vi "Send NEA_Get Data.vi"(7 "Message Priority (Normal)":T2=enum."Normal", 8 "error in (no error)":errorcluster, 10 "Data":T1={"M2 Dataset"={"Read Temp"=273.15, "Feedback"=1, "Set Temp"=273.15}, "M1 Dataset"={"Read Temp"=273.15, "Feedback"=1, "Set Temp"=273.15}, "Comp"=FALSE} {"M1 Dataset"."Set Temp" format="%.1f"; "M1 Dataset"."Feedback" items=["Evap Temp", "Case Temp", "Intec Temp", "TSD  Temp", "Autotune", "Extra"]; "M1 Dataset"."Read Temp" format="%.1f"; "M2 Dataset"."Set Temp" format="%.1f"; "M2 Dataset"."Feedback" items=["Evap Temp", "Case Temp", "Intec Temp", "TSD  Temp", "Autotune", "Extra"]; "M2 Dataset"."Read Temp" format="%.1f"}, 11 "Message Enqueuer":refnum<class "Message Enqueuer.lvclass">) -> (0 "error out":errorcluster, 3 "Message Enqueuer out":refnum<class "Message Enqueuer.lvclass">)   [LabVIEW 2019, in "Test.lvlib" / "NEA_Get Data Msg.lvclass"]
doc: "This VI sends the message to an actor."
uses:
  NEA_Get Data Msg.lvclass
  <vilib>/ActorFramework/Message Enqueuer/Message Enqueuer.lvclass
  <vilib>/ActorFramework/Message Enqueuer/Message Priority.ctl
  Type Defs/Cobra Data.ctl
  C:/Program Files (x86)/National Instruments/LabVIEW 2019/vi.lib/ActorFramework/Message/Message.lvclass
  NEA_Get Data Msg.lvclass/NEA_Get Data Msg.ctl
  <vilib>/ActorFramework/Message Enqueuer/Message Enqueuer.lvclass/Message Enqueuer.ctl
  <vilib>/ActorFramework/Message Priority Queue/Priority Enqueue.vi
  Test.lvlib
panel:
  # "degC"
  # "degC"
  # "degC"
  # "degC"
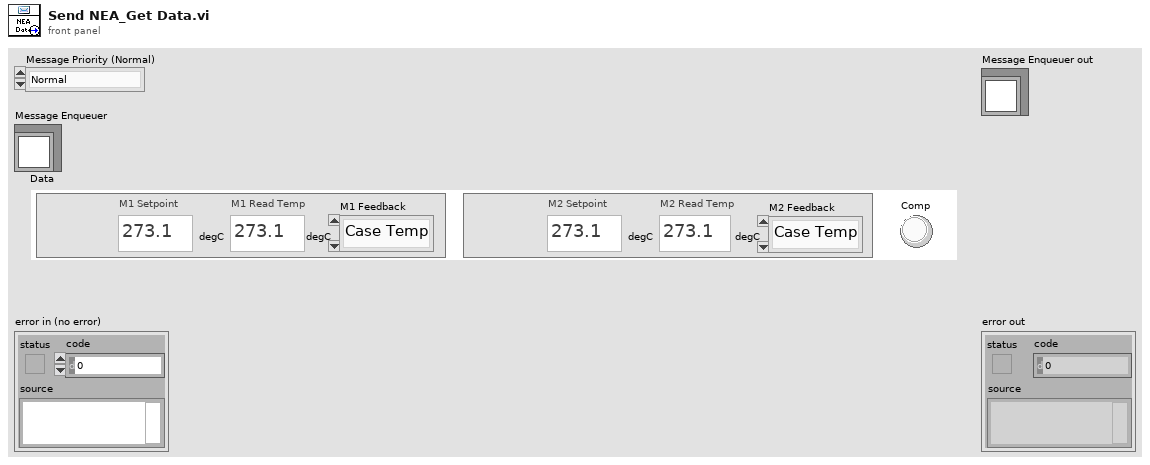
[diagram p1: front panel]
types:
  T1 = typedef "Test.lvlib/Cobra Data.ctl" = cluster{"M2 Dataset":cluster{"Read Temp":dbl, "Feedback":u8, "Set Temp":dbl}, "M1 Dataset":cluster{"Read Temp":dbl, "Feedback":u8, "Set Temp":dbl}, "Comp":bool}
  T2 = typedef "Actor Framework.lvlib/Message Enqueuer.lvclass/Message Priority.ctl" = enum16{"Low", "Normal", "High"}
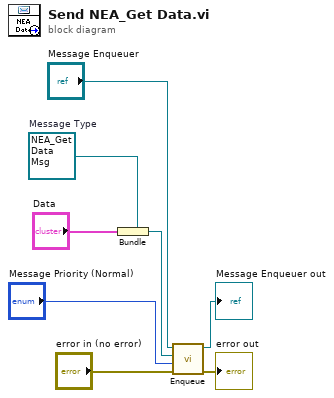
[diagram p0: block diagram]
diagram:
  w5 = refnum<class "NEA_Get Data Msg.lvclass"> refnum  # Message Type
  n1 = Bundle(cluster=w5, "Data") -> (w4:refnum<class "NEA_Get Data Msg.lvclass">)
  n2 = call <vilib>:"Enqueue.vi"("error in (no error)"="error in (no error)", "Message Priority (Normal)"="Message Priority (Normal)", "Message"=w4, "Message Enqueuer in"="Message Enqueuer") -> ("error out"=→"error out":errorcluster, "Message Enqueuer out"=→"Message Enqueuer out":refnum<class "Message Enqueuer.lvclass">)  [unwired: 6 in]
